vi "Read_Write_Template.vi"(0 "Template File":path, 1 "Mode":T1, 5 "Channel names In":string[](array[string]), 7 "Single Value In":string, 9 "2D Info In":string[][](array[string]), 11 "1D Info In":string[](array[string]), 12 "Save file":bool=TRUE, 13 "Data type":string="Tolerance") -> (2 "Valid Template File?":bool, 3 "Freshly Loaded?":bool, 4 "Template File Out":path, 6 "Template Ch Names Out":string[](array[string]), 8 "Single Value Out":string, 10 "2D Info Out":string[][](array[string]), 14 "Template Info":string[][](array[string]), 15 "1D Info Out":string[](array[string]))   [LabVIEW 2022 SP3]
uses:
  Controls/Global_mode.ctl
  Results_plotter_Global.vi
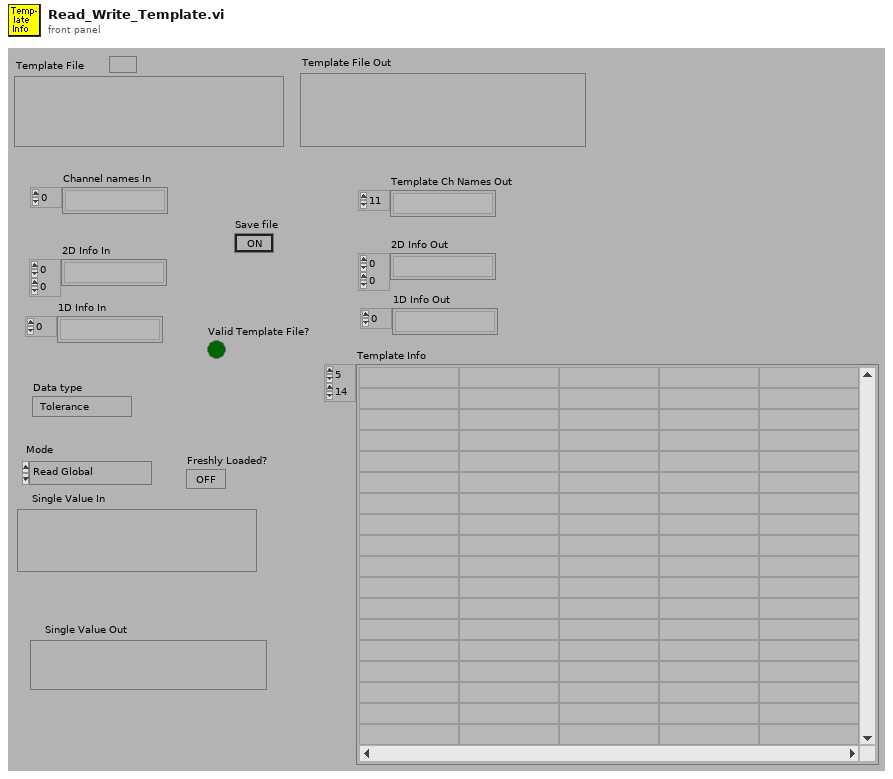
[diagram p1: front panel]
types:
  T1 = typedef "Global_mode.ctl" = enum16{"Read Global", "Load Global From File", "Write Global to File"}
  T2 = typedef "File_Status.ctl" = enum16{"Invalid Path", "File Does not Exist", "This is a folder pathname", "Generic File Error", "Directory structure cannot be created", "File cannot be created", "File can be created", "File exist but read only", "File exist but no access", "File exist with read and write access"}
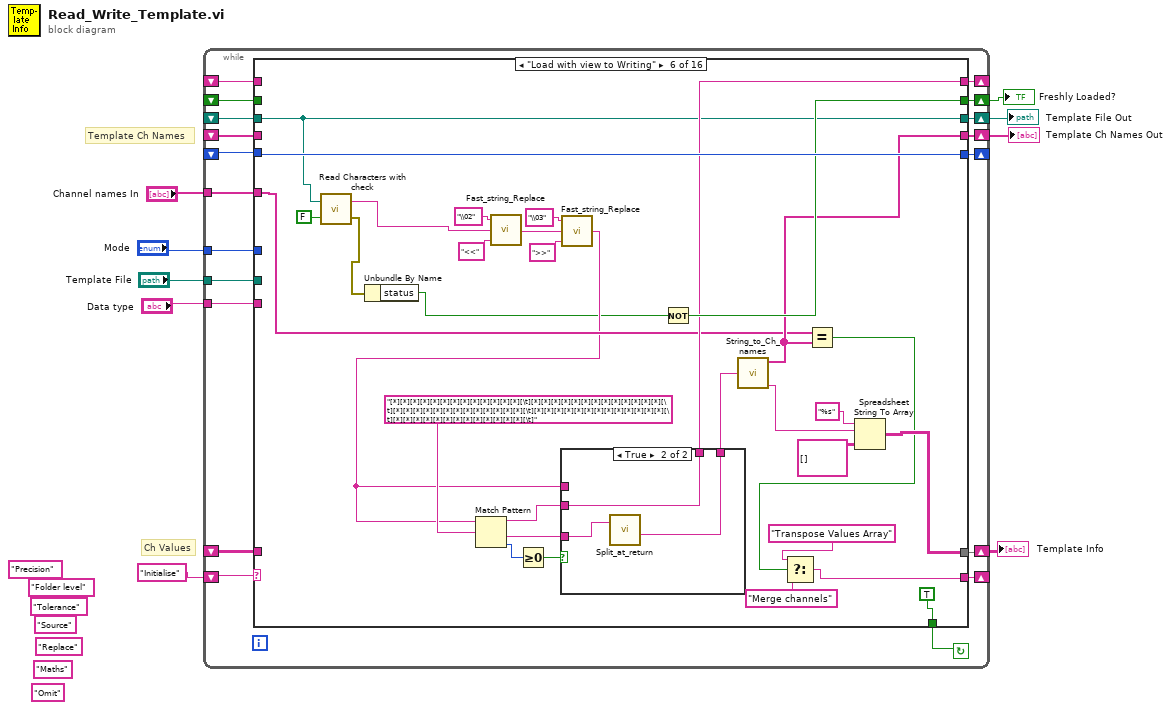
[diagram p0: block diagram]
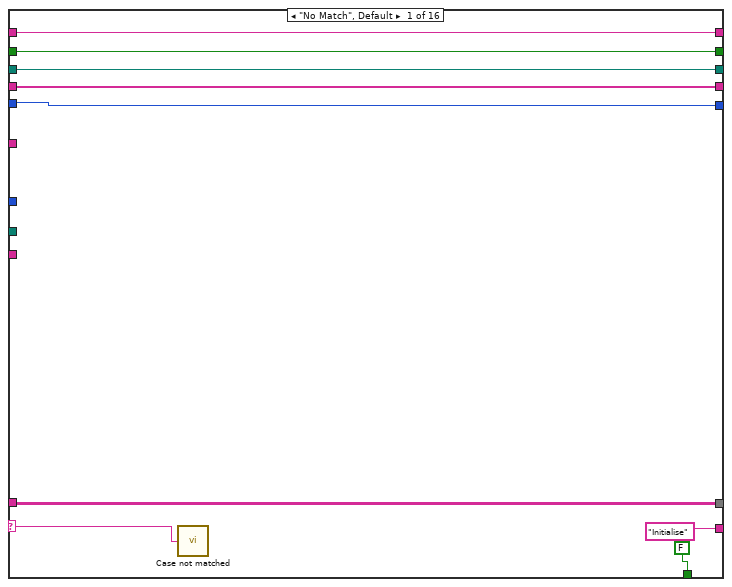
[diagram p2: hidden frame]
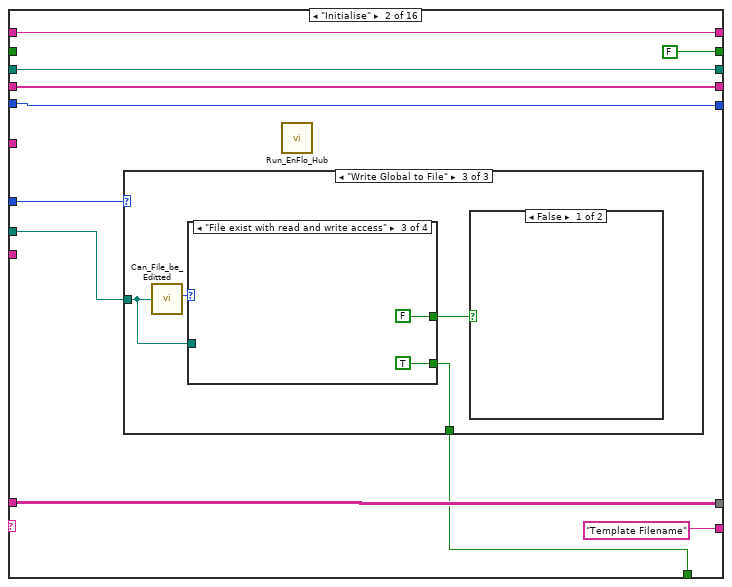
[diagram p3: hidden frame]
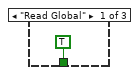
[diagram p4: hidden frame]
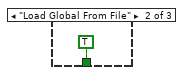
[diagram p5: hidden frame]
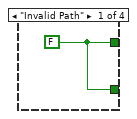
[diagram p6: hidden frame]
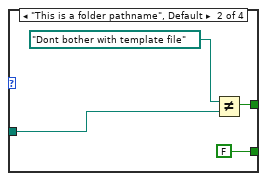
[diagram p7: hidden frame]
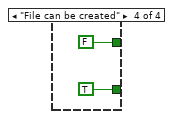
[diagram p8: hidden frame]
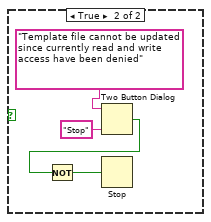
[diagram p9: hidden frame]
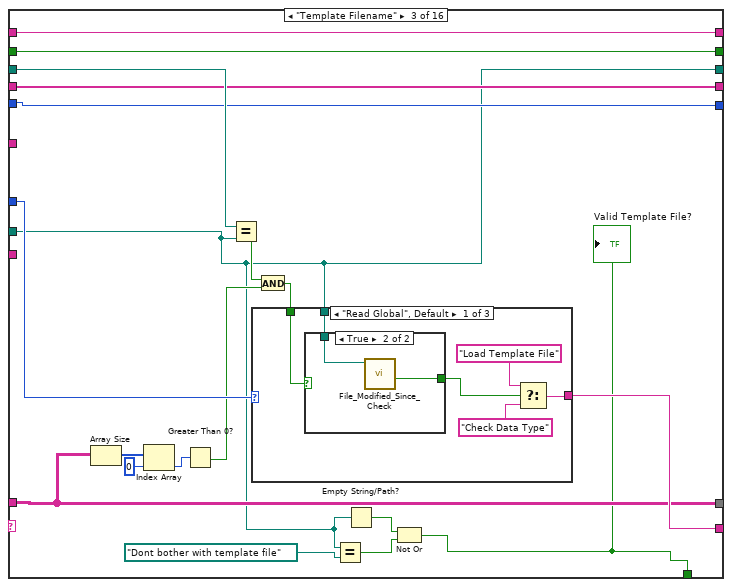
[diagram p10: hidden frame]
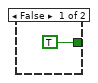
[diagram p11: hidden frame]
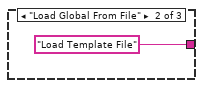
[diagram p12: hidden frame]
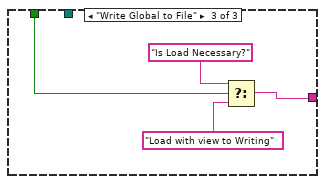
[diagram p13: hidden frame]
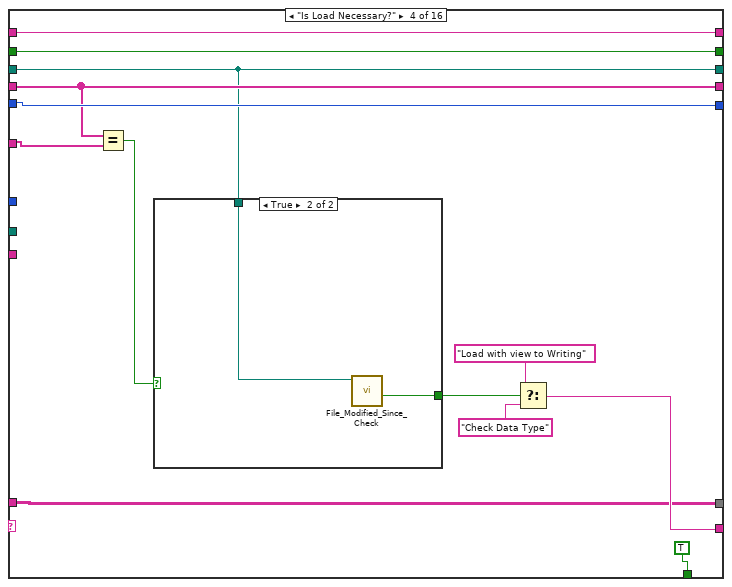
[diagram p14: hidden frame]
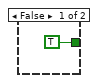
[diagram p15: hidden frame]
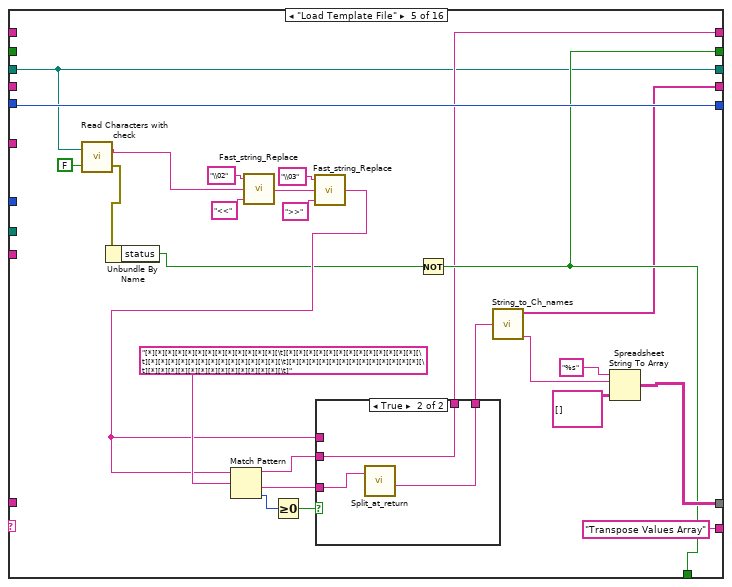
[diagram p16: hidden frame]
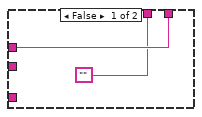
[diagram p17: hidden frame]
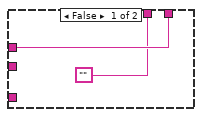
[diagram p18: hidden frame]
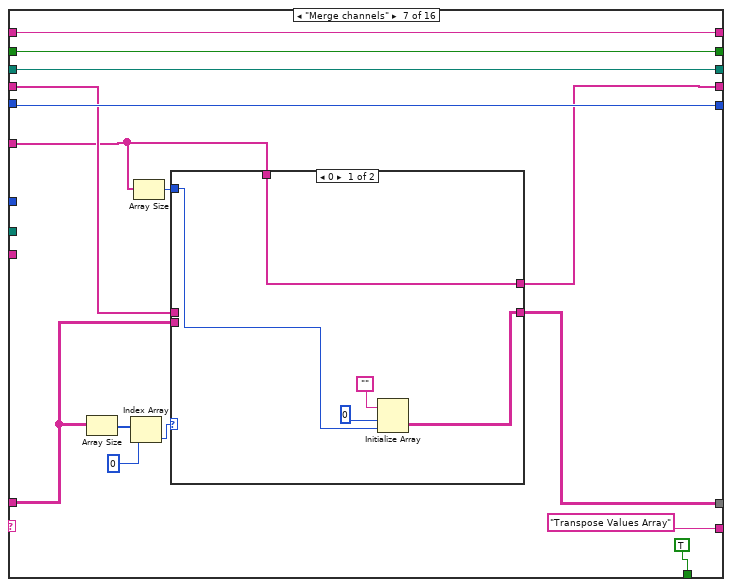
[diagram p19: hidden frame]
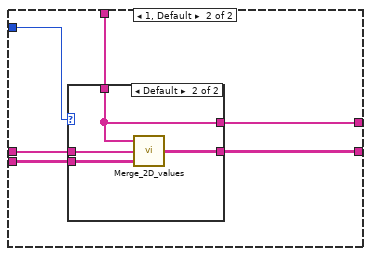
[diagram p20: hidden frame]
diagram:
  (unwired) "Precision"
  (unwired) "Folder level"
  (unwired) "Omit"
  (unwired) "Maths"
  (unwired) "Tolerance"
  (unwired) "Source"
  (unwired) "Replace"
  # "Template Ch Names"
  # "Ch Values"
  n1 = while {
    shift-left: _ -> [w13]
    shift-right: [w14] -> w2
    tunnel: "Channel names In" -> [w16]
    shift-left: _ -> [w15]
    shift-right: [w17] -> _
    tunnel: "Data type" -> [w18]
    shift-left: _ -> [w19]
    shift-right: [w20] -> w5
    shift-left: _ -> [w23]
    shift-right: [w22] -> w6
    shift-left: _ -> [w24]
    shift-right: [w25] -> w7
    tunnel: "Mode" -> [w26]
    shift-left: "Initialise" -> [w21]
    shift-right: [w27] -> _
    shift-right: [w12] -> _
    shift-left: _ -> [w11]
    tunnel: "Template File" -> [w10]
    stop <- w28 continue-if-true
    n2 = case shown="\"Load with view to Writing\"" w21 {
      selector: w21 -> [w29 _ _ _ _ _ _ _ _ _ _ _ _ _ _ _]
      tunnel: [FALSE w38 w68 TRUE w135 TRUE ("Save file") TRUE ("Save file") TRUE w238 FALSE FALSE FALSE "Save file" TRUE ("Save file") w452 FALSE] -> w28
      tunnel: ["Initialise" "Template Filename" w82 w112 "Transpose Values Array" w160 "Transpose Values Array" "Check Data Type" w235 "" "" "" "Save Template File" "Save Template File" w449 "End"] -> w27
      tunnel: w26 -> [_ w40 w83 _ _ _ _ _ w237 _ _ _ _ _ _ _]
      tunnel: [w34 w46 w78 w106 w139 w176 w191 w225 w241 w295 w309 w329 w355 w438 w447 w498] -> w25
      tunnel: w24 -> [w34 w46 w78 w106 _ _ w189 w224 w241 w295 w309 w329 w356 w438 w446 w498]
      tunnel: w23 -> [w36 w47 w85 w102 w119 w150 w193 w220 w240 w297 w315 w331 w357 w433 w451 w490]
      tunnel: [w36 w47 w67 w102 w119 w150 w193 w220 w240 w297 w315 w331 w357 w433 w451 w490] -> w22
      tunnel: [w37 w45 w84 w105 w127 w164 w184 w219 w239 w293 w310 w326 w350 w441 w450 w497] -> w20
      tunnel: w19 -> [w37 w45 w84 w105 _ _ w192 w219 w239 w293 w310 w326 w350 w441 w450 w497]
      tunnel: w18 -> [_ _ _ _ _ _ _ _ w242 w296 w307 w330 w353 w434 _ _]
      tunnel: [w32 w43 w77 w110 w140 w177 w196 w218 w236 w286 w312 w318 w348 w440 w448 w495] -> w17
      tunnel: w16 -> [_ _ _ w104 _ w163 w183 _ _ w287 _ w323 w349 _ _ _]
      tunnel: w15 -> [w32 w43 w77 w110 w140 w177 w196 w218 _ w286 w312 w318 w348 w440 w448 w495]
      tunnel: [w31 FALSE w73 w101 w135 w172 w194 w216 w234 w285 w311 w317 w347 w439 w445 w494] -> w14
      tunnel: w13 -> [w31 _ w73 w101 _ _ w194 w216 w234 w285 w311 w317 w347 w439 w445 w494]
      tunnel: [w30 w41 w72 w100 w129 w166 w195 w215 w233 w284 w308 w316 w345 w436 w443 w493] -> w12
      tunnel: w11 -> [w30 w41 w72 w100 _ _ w195 w215 w233 w284 w308 w316 w345 w435 w444 w493]
      tunnel: w10 -> [_ w39 w67 _ _ _ _ _ _ _ _ _ _ _ _ _]
      frame "No Match", Default {
        n3 = call "Case not matched.vi"("Case Name not Matched"=w29) -> ()
      }
      frame "Initialise" {
        n4 = case shown="\"Write Global to File\"" w40 {
          tunnel: w39 -> [_ _ w50]
          tunnel: [TRUE TRUE w51] -> w38
          frame "Read Global" {
          }
          frame "Load Global From File" {
          }
          frame "Write Global to File" {
            n5 = call "Can_File_be_Editted.vi"("Filename"=w50) -> ("File Status"=w53:T2)  [unwired: 3 out]
            n6 = case shown="\"File exist with read and write access\"" w53 {
              tunnel: [w54 w56 FALSE FALSE] -> w52
              tunnel: [w54 FALSE TRUE TRUE] -> w51
              tunnel: w50 -> [_ w55 _ _]
              frame "Invalid Path" {
                w54 = FALSE
              }
              frame "This is a folder pathname", Default {
                n7 = Not Equal?(x=path "Dont bother with template file" ("Template File"), y=w55) -> (x != y?=w56:bool)
              }
              frame "File exist with read and write access" {
              }
              frame "File can be created" {
              }
            }
            n8 = case shown="False" w52 {
              frame False {
              }
              frame True {
                n9 = Two Button Dialog(message="Template file cannot be updated since currently read and write access have been denied", 1:"Stop" ("F button name (\"Cancel\")")) -> (T button?=w64:bool)  [unwired: 1 out]
                n10 = Not(x=w64) -> (.not. x?=w63:bool)
                n11 = Stop(stop? (T)=w63) -> ()
              }
            }
          }
        }
        n12 = call "Run_EnFlo_Hub.vi"() -> ()  [unwired: 1 in, 7 out]
      }
      frame "Template Filename" {
        n13 = Array Size(array=w78) -> (size(s)=w79:i32[])
        n14 = Index Array(array=w79, index=0 ("Index")) -> (element=w81:i32)
        n15 = Greater Than 0?(x=w81) -> (x > 0?=w74:bool)
        n16 = Equal?(x=w85, y=w67) -> (x = y?=w76:bool)
        n17 = And(x=w76, y=w74) -> (x .and. y?=w75:bool)
        n18 = case shown="\"Read Global\", Default" w83 {
          tunnel: w75 -> [w91 _ w99]
          tunnel: [w87 "Load Template File" w97] -> w82
          tunnel: w67 -> [w90 _ _]
          frame "Read Global", Default {
            n19 = case shown="True" w91 {
              tunnel: w90 -> [_ w94]
              tunnel: [TRUE ("Modified?") w93] -> w89
              frame False {
              }
              frame True {
                n20 = call "File_Modified_Since_Check.vi"("File Path"=w94) -> ("modifiedSinceRead"=w93:bool)  [unwired: 7 in, 1 out]
              }
            }
            n21 = Select(t="Load Template File", s=w89, f="Check Data Type") -> (s? t:f=w87:string)
          }
          frame "Load Global From File" {
          }
          frame "Write Global to File" {
            n22 = Select(t="Is Load Necessary?", s=w99, f="Load with view to Writing") -> (s? t:f=w97:string)
          }
        }
        n23 = Equal?(x=w67, y=path "Dont bother with template file" ("Template File")) -> (x = y?=w70:bool)
        n24 = Empty String/Path?(string/path=w67) -> (empty?=w69:bool)
        n25 = Not Or(1:w70, 2:w69) -> (0:w68:bool)
        "Valid Template File?" <- w68
      }
      frame "Is Load Necessary?" {
        n26 = Equal?(x=w105, y=w104) -> (x = y?=w103:bool)
        n27 = case shown="True" w103 {
          tunnel: w102 -> [_ w115]
          tunnel: [TRUE ("Modified?") w114] -> w109
          frame False {
          }
          frame True {
            n28 = call "File_Modified_Since_Check.vi"("File Path"=w115) -> ("modifiedSinceRead"=w114:bool)  [unwired: 7 in, 1 out]
          }
        }
        n29 = Select(t="Load with view to Writing", s=w109, f="Check Data Type") -> (s? t:f=w112:string)
      }
      frame "Load Template File" {
        n30 = call "Read Characters with check.vi"("Call EnFlo Error Handler?"=FALSE, "file (use dialog)"=w119) -> ("error out"=w117:errorcluster, "Read String"=w118:string)
        n31 = Unbundle By Name(w117) -> ("status"=w120:bool)
        n32 = call "Fast_string_Replace.vi"("Replace match with:"="<<" ("regular expression"), "Input String"=w118, "regular expression"="\\02") -> ("Output String"=w121:string)  [unwired: 2 out]
        n33 = call "Fast_string_Replace.vi"("Replace match with:"=">>" ("regular expression"), "Input String"=w121, "regular expression"="\\03") -> ("Output String"=w126:string)  [unwired: 2 out]
        n34 = Match Pattern(string=w126, regular expression="[*][*][*][*][*][*][*][*][*][*][*][*][*][\t][*][*][*][*][*][*][*][*][*][*][*][*][*][\t][*][*][*][*][*][*][*][*][*][*][*][*][*][\t][*][*][*][*][*][*][*][*][*][*][*][*][*][\t][*][*][*][*][*][*][*][*][*][*][*][*][*][\t]" ("String")) -> (before substring=w128:string, after substring=w133:string, offset past match=w132:i32)  [unwired: 2 out]
        n35 = Greater Or Equal To 0?(x=w132) -> (x >= 0?=w131:bool)
        n36 = case shown="True" w131 {
          tunnel: w133 -> [_ w146]
          tunnel: [w143 w145] -> w130
          tunnel: w126 -> [w143 _]
          tunnel: ["" w144] -> w129
          tunnel: w128 -> [_ w144]
          frame False {
          }
          frame True {
            n37 = call "Split_at_return.vi"("String"=w146) -> ("after substring"=w145:string)  [unwired: 1 in, 3 out]
          }
        }
        n38 = Not(x=w120) -> (.not. x?=w135:bool)
        n39 = call "String_to_Ch_names.vi"("Spreadsheet string"=w130) -> ("Ch names"=w127:string[], "String After names"=w136:string)  [unwired: 2 out]
        n40 = Spreadsheet String To Array(format string="%s", spreadsheet string=w136, array type (2D Dbl)=string[][] [] ("Channel Values")) -> (array=w139:string[][])  [unwired: 1 out]
      }
      frame "Load with view to Writing" {
        n41 = call "Read Characters with check.vi"("Call EnFlo Error Handler?"=FALSE, "file (use dialog)"=w150) -> ("error out"=w148:errorcluster, "Read String"=w149:string)
        n42 = Unbundle By Name(w148) -> ("status"=w151:bool)
        n43 = call "Fast_string_Replace.vi"("Replace match with:"="<<" ("regular expression"), "Input String"=w149, "regular expression"="\\02") -> ("Output String"=w153:string)  [unwired: 2 out]
        n44 = call "Fast_string_Replace.vi"("Replace match with:"=">>" ("regular expression"), "Input String"=w153, "regular expression"="\\03") -> ("Output String"=w152:string)  [unwired: 2 out]
        n45 = Match Pattern(string=w152, regular expression="[*][*][*][*][*][*][*][*][*][*][*][*][*][\t][*][*][*][*][*][*][*][*][*][*][*][*][*][\t][*][*][*][*][*][*][*][*][*][*][*][*][*][\t][*][*][*][*][*][*][*][*][*][*][*][*][*][\t][*][*][*][*][*][*][*][*][*][*][*][*][*][\t]" ("String")) -> (before substring=w165:string, after substring=w170:string, offset past match=w169:i32)  [unwired: 2 out]
        n46 = Greater Or Equal To 0?(x=w169) -> (x >= 0?=w168:bool)
        n47 = case shown="True" w168 {
          tunnel: w170 -> [_ w182]
          tunnel: [w179 w181] -> w167
          tunnel: w152 -> [w179 _]
          tunnel: ["" w180] -> w166
          tunnel: w165 -> [_ w180]
          frame False {
          }
          frame True {
            n48 = call "Split_at_return.vi"("String"=w182) -> ("after substring"=w181:string)  [unwired: 1 in, 3 out]
          }
        }
        n49 = Not(x=w151) -> (.not. x?=w172:bool)
        n50 = call "String_to_Ch_names.vi"("Spreadsheet string"=w167) -> ("Ch names"=w164:string[], "String After names"=w173:string)  [unwired: 2 out]
        n51 = Equal?(x=w163, y=w164) -> (x = y?=w162:bool)
        n52 = Select(t="Transpose Values Array", s=w162, f="Merge channels") -> (s? t:f=w160:string)
        n53 = Spreadsheet String To Array(format string="%s", spreadsheet string=w173, array type (2D Dbl)=string[][] [] ("Channel Values")) -> (array=w176:string[][])  [unwired: 1 out]
      }
      frame "Merge channels" {
        n54 = Array Size(array=w189) -> (size(s)=w188:i32[])
        n55 = Index Array(array=w188, index=0) -> (element=w186:i32)
        n56 = Array Size(array=w183) -> (size(s)=w185:i32)
        n57 = case shown="0" w186 {
          tunnel: w183 -> [w198 w208]
          tunnel: w192 -> [_ w207]
          tunnel: w189 -> [_ w206]
          tunnel: [w200 w205] -> w191
          tunnel: w185 -> [w199 w204]
          tunnel: [w198 w203] -> w184
          frame 0 {
            n58 = Initialize Array("", 0 ("Dimension Size"), w199) -> (w200:string[][])
          }
          frame 1, Default {
            n59 = case shown="Default" w204 {
              tunnel: w208 -> [_ w211]
              tunnel: w207 -> [w210 w214]
              tunnel: w206 -> [w209 w213]
              tunnel: [w209 w212] -> w205
              tunnel: [w210 w211] -> w203
              frame 0 {
              }
              frame Default {
                n60 = call "Merge_2D_values.vi"("Values In"=w213, "Present Channels"=w214, "Desired Channels"=w211) -> ("Values Out"=w212:string[][])
              }
            }
          }
        }
      }
      frame "Transpose Values Array" {
        n61 = Array Size(array=w224) -> (size(s)=w222:i32[])
        n62 = Index Array(array=w222, index=1 ("Index")) -> (element=w221:i32)
        n63 = for {
          N: w221 -> [_]
          tunnel: w224 -> [w229]
          tunnel: [w230] -> w225 mode=indexing
          i -> [w228]
          n64 = Index Array(array=w229, index (col)=w228) -> (element=w227:string[])  [unwired: 1 in]
          n65 = for {
            tunnel: [w232] -> w230 mode=indexing
            tunnel: w227 -> [w231] mode=indexing
            n66 = call "Remove_Quotes.vi"("String"=w231) -> ("String Out"=w232:string)
          }
        }
      }
      frame "Check Data Type" {
        n67 = case shown="\"Replace\"" w242 {
          tunnel: [1 1 1 1 2 1 1 2 2 2 1 2 1 1 1 0] -> w236
          tunnel: w242 -> [_ _ _ _ _ _ _ _ _ _ _ _ _ _ _ _]
          tunnel: [TRUE TRUE TRUE TRUE TRUE TRUE TRUE TRUE TRUE TRUE TRUE TRUE TRUE TRUE TRUE TRUE] -> w238
          frame "Description" {
          }
          frame "Dispose" {
          }
          frame "Decimal" {
          }
          frame "Precision" {
          }
          frame "Multiple Sources" {
          }
          frame "Summarise" {
          }
          frame "Tolerance" {
          }
          frame "Source" {
          }
          frame "Replace" {
          }
          frame "Ignore When" {
          }
          frame "Maths" {
          }
          frame "Omit" {
          }
          frame "Folder level" {
          }
          frame "Minimum Value" {
          }
          frame "Maximum Value" {
          }
          frame "Log Folder Name", Default {
          }
        }
        n68 = case shown="\"Read Global\", Default" w237 {
          tunnel: w236 -> [w244 w248]
          tunnel: [w243 w249] -> w235
          frame "Read Global", Default {
            n69 = case shown="2, Default" w244 {
              tunnel: ["Create Outputs 2D" "Create Outputs 1D" "Create single value output"] -> w243
              frame 2, Default {
              }
              frame 1 {
              }
              frame 0 {
              }
            }
          }
          frame "Write Global to File" {
            n70 = case shown="0" w248 {
              tunnel: ["Replace single value" "Replace Values"] -> w249
              frame 0 {
              }
              frame 1, Default {
              }
            }
          }
        }
      }
      frame "Create Outputs 1D" {
        n71 = for {
          tunnel: w296 -> [w305]
          tunnel: w295 -> [w304] mode=indexing
          tunnel: [w303] -> w294 mode=indexing
          n72 = call "Get_Array_Subset.vi"("String Array In"=w304, "Subset Name"=w305) -> ("First Element"=w303:string)  [unwired: 4 out]
        }
        n73 = Array Size(array=w287) -> (size(s)=w289:i32)
        n74 = Equal To 0?(x=w289) -> (x = 0?=w288:bool)
        n75 = case shown="True" w288 {
          tunnel: w294 -> [w301 w302]
          tunnel: w287 -> [w300 _]
          tunnel: w293 -> [w299 _]
          tunnel: [w298 w302] -> w292
          frame False {
            n76 = call "Merge_row_values.vi"("Present Row values"=w301, "Present Channels"=w299, "Desired Channels"=w300) -> ("Desired Row values"=w298:string[])  [unwired: 1 out]
          }
          frame True {
          }
        }
        "1D Info Out" <- w292
      }
      frame "Create single value output" {
        n77 = call "Get_Characters_from_string.vi"("Input string"=w308, "Variable name"=w307) -> ("Value"=→"Single Value Out":string)  [unwired: 1 in, 1 out]
      }
      frame "Create Outputs 2D" {
        n78 = for {
          tunnel: w330 -> [w344]
          tunnel: w329 -> [w343] mode=indexing
          tunnel: [w342] -> w325 mode=indexing
          n79 = call "Get_Array_Subset.vi"("String Array In"=w343, "Subset Name"=w344) -> ("Array Subset Out"=w342:string[])  [unwired: 4 out]
        }
        n80 = Equal?(x=w326, y=w323) -> (x = y?=w321:bool)
        n81 = Array Size(array=w323) -> (size(s)=w322:i32)
        n82 = Equal To 0?(x=w322) -> (x = 0?=w320:bool)
        n83 = Or(x=w321, y=w320) -> (x .or. y?=w319:bool)
        n84 = case shown="False" w319 {
          tunnel: w326 -> [w335 _]
          tunnel: w323 -> [w334 _]
          tunnel: w325 -> [w333 w341]
          tunnel: [w332 w341] -> w324
          frame False {
            n85 = for {
              tunnel: w335 -> [w340]
              tunnel: w334 -> [w339] mode=indexing
              tunnel: w333 -> [w337]
              tunnel: [w336] -> w332 mode=indexing
              workers-P: _ -> [_]
              n86 = Search 1D Array(1D array=w340, element=w339) -> (index of element=w338:i32)  [unwired: 1 out]
              n87 = Index Array(array=w337, index (row)=w338) -> (element=w336:string[])  [unwired: 1 in]
            }
          }
          frame True {
          }
        }
        "2D Info Out" <- w324
      }
      frame "Replace Values" {
        n88 = for {
          tunnel: w353 -> [w366]
          tunnel: w356 -> [w365] mode=indexing
          tunnel: [w364] -> w355 mode=indexing
          tunnel: w350 -> [w363] mode=indexing
          tunnel: w348 -> [w362]
          tunnel: "1D Info In" -> [w361]
          tunnel: "2D Info In" -> [w360]
          tunnel: w350 -> [w359] mode=indexing
          tunnel: w349 -> [w358]
          n89 = stacked-sequence {
            seq-local: [_ w376 _ _ _] -> [_ _ _ w427 _]
            seq-local: [_ w375 _ _ _] -> [_ _ _ w428 _]
            seq-local: [_ _ w387 _ _] -> [_ _ _ w426 _]
            seq-local: [_ w374 _ _ _] -> [_ _ w383 _ _]
            seq-local: [w369 _ _ _ _] -> [_ _ w384 _ _]
            seq-local: [w367 _ _ _ _] -> [_ _ w382 _ _]
            tunnel: w366 -> [_ w381 _ w429 _]
            tunnel: w365 -> [_ w378 _ _ _]
            tunnel: [_ _ _ w419 _] -> w364
            tunnel: w363 -> [_ _ _ w420 _]
            tunnel: w362 -> [w368 _ _ _ _]
            tunnel: w361 -> [_ _ w386 _ _]
            tunnel: w360 -> [_ _ w385 _ _]
            tunnel: w359 -> [w371 _ _ _ _]
            tunnel: w358 -> [w370 _ _ _ _]
            frame #0 {
              n90 = Search 1D Array(1D array=w370, element=w371) -> (index of element=w367:i32)  [unwired: 1 out]
              n91 = case shown="0, Default" w367 {
                tunnel: [w372 0] -> w369
                tunnel: w368 -> [w372 _]
                frame 0, Default {
                }
                frame -1 {
                }
              }
            }
            frame #1 {
              n92 = call "Get_Array_Subset.vi"("String Array In"=w378, "Subset Name"=w381) -> ("index after match"=w377:i32, "Array Subset Out"=w374:string[], "Length before match"=w379:i32)  [unwired: 2 out]
              n93 = Array Subset(array=w378, index=0 ("Array Index"), length=w379) -> (w376:string[])
              n94 = Array Subset(array=w378, index=w377) -> (w375:string[])  [unwired: 1 in]
            }
            frame #2 {
              n95 = case shown="2, Default" w384 {
                tunnel: [w391 w415 w418] -> w387
                tunnel: w386 -> [_ w417 _]
                tunnel: w385 -> [w390 _ _]
                tunnel: w383 -> [_ _ w418]
                tunnel: w382 -> [w388 w414 _]
                frame 2, Default {
                  n96 = Index Array(array=w390, index (row)=w388) -> (element=w389:string[])  [unwired: 1 in]
                  n97 = while {
                    shift-left: _ -> [w392]
                    shift-right: [w393] -> _
                    tunnel: [w394] -> w391
                    tunnel: w389 -> [w396]
                    i -> [w397]
                    stop <- w395 continue-if-true
                    n98 = case shown="0, Default" w397 {
                      tunnel: w396 -> [w399 w402]
                      tunnel: [w400 FALSE] -> w395
                      tunnel: [w399 w405] -> w394
                      tunnel: [w398 w404] -> w393
                      tunnel: w392 -> [_ w404]
                      frame 0, Default {
                        n99 = Empty String/Path?(string/path=w399) -> (empty?=w398:bool[])
                        n100 = Or Array Elements(Boolean array=w398) -> (logical OR=w400:bool)
                      }
                      frame 1 {
                        n101 = for {
                          shift-right: [w408] -> w405
                          shift-left: string[] [] -> [w407]
                          tunnel: w404 -> [w409] mode=indexing
                          tunnel: w402 -> [w406] mode=indexing
                          n102 = case shown="True" w409 {
                            tunnel: [w411 w413] -> w408
                            tunnel: w407 -> [w412 w413]
                            tunnel: w406 -> [w410 _]
                            frame False {
                              n103 = Build Array (concatenate)(w412, w410) -> (w411:string[])
                            }
                            frame True {
                            }
                          }
                        }
                      }
                    }
                  }
                }
                frame 1 {
                  n104 = Index Array(array=w417, index=w414) -> (element=w416:string)
                  n105 = Build Array(w416) -> (w415:string[])
                }
                frame 0 {
                }
              }
            }
            frame #3 {
              w421 = ""
              n106 = Format Into String(format string="**%s Start**" ("Format String"), w429) -> (resulting string=w425:string)  [unwired: 2 in, 1 out]
              n107 = Format Into String(format string="**%s End**" ("Format String"), w429) -> (resulting string=w424:string)  [unwired: 2 in, 1 out]
              n108 = Build Array (concatenate)(w427, w425, w426, w424, w428) -> (w423:string[])
              n109 = call "Clean_Up_Template.vi"("Template Info In"=w423) -> ("Template Info Out"=w422:string[])
              n110 = Build Array (concatenate)(w421, w420, w421, w422) -> (w419:string[])
            }
            frame #4 {
            }
          }
        }
      }
      frame "Replace single value" {
        n111 = call "Replace_data_in_setup_string.vi"("New data string"="Single Value In", "Input string"=w435, "Variable name"=w434) -> ("Appended string"=w436:string)
      }
      frame "Save Template File" {
        n112 = stacked-sequence {
          seq-local: [w455 _] -> [_ w468]
          tunnel: [_ TRUE] -> w452
          tunnel: w451 -> [_ w478]
          tunnel: w450 -> [_ w477]
          tunnel: [_ "Update last Modified VI"] -> w449
          tunnel: [_ w471] -> w447
          tunnel: w446 -> [_ w470]
          tunnel: w444 -> [w454 _]
          tunnel: [w453 _] -> w443
          frame #0 {
            w460 = "Log Folder Name" ("Variable name")
            n113 = call "Get_Characters_from_string.vi"("Input string"=w454, "Variable name"=w460) -> ("Status"=w461:enum16{"Char in string", "Char not in string"})  [unwired: 1 in, 1 out]
            n114 = case shown="\"Char not in string\"" w461 {
              tunnel: w460 -> [_ w467]
              tunnel: w454 -> [w462 w464]
              tunnel: [w462 w463] -> w453
              frame "Char in string" {
              }
              frame "Char not in string" {
                n115 = Default Directory() -> (w466:path)
                n116 = Path To String(path=w466) -> (string=w465:string)
                n117 = call "Characters_to_string.vi"("stringIn"=w464, "Characters to write"=w465, "Label for characters"=w467) -> ("Output string"=w463:string)
              }
            }
            n118 = Initialize Array("", 10 ("Dimension Size")) -> (w459:string[])
            n119 = call "Asterisk_header.vi"("Channel names"=w459) -> ("Header string"=w456:string)
            n120 = Concatenate Strings(w453, w456) -> (w455:string)
          }
          frame #1 {
            w476 = FALSE  # exists?
            n121 = Transpose 2D Array(2D array=w470) -> (transposed array=w474:string[][])
            n122 = for {
              shift-right: [w481] -> w472
              shift-left: string[][] [] -> [w480]
              tunnel: w474 -> [w479] mode=indexing
              n123 = Equal?(x=w479, y=" ") -> (x = y?=w483:bool[])
              n124 = And Array Elements(Boolean array=w483) -> (logical AND=w482:bool)
              n125 = case shown="False" w482 {
                tunnel: [w486 w488] -> w481
                tunnel: w480 -> [w487 w488]
                tunnel: w479 -> [w485 _]
                frame False {
                  n126 = Build Array (concatenate)(w487, w485) -> (w486:string[][])
                }
                frame True {
                }
              }
            }
            n127 = Transpose 2D Array(2D array=w472) -> (transposed array=w471:string[][])
            n128 = call "Write_Ch_data_file.vi"("Header string"=w468, "exists?"=w476, "Channel Values"=w472, "Channel names"=w477, "Filename"=w478) -> ()  [unwired: 2 in, 5 out]
          }
        }
      }
      frame "Update last Modified VI" {
        n129 = global read "Results_plotter_Global.vi" "Load number"() -> (w491:i32)
        n130 = call "File_Modified_Since_Check.vi"("mode"="File just Read", "File Path"=w490) -> ()  [unwired: 6 in, 2 out]
        n131 = Increment(x=w491) -> (x+1=w492:i32)
        n132 = global write "Results_plotter_Global.vi" "Load number"(w492) -> ()
      }
    }
  }
  "Template Ch Names Out" <- w5
  "Template File Out" <- w6
  "Template Info" <- w7
  "Freshly Loaded?" <- w2
